vi "LakeShore218_01_Main.vi"() -> ()   [LabVIEW 2019]
uses:
  LakeShore218_Global.vi
panel:
  in  "onoff_ch8":enum16{"Off", "On"}(ring)
  in  "onoff_ch7":enum16{"Off", "On"}(ring)
  in  "onoff_ch6":enum16{"Off", "On"}(ring)
  in  "onoff_ch5":enum16{"Off", "On"}(ring)
  in  "onoff_ch4":enum16{"Off", "On"}(ring)
  in  "onoff_ch3":enum16{"Off", "On"}(ring)
  in  "onoff_ch2":enum16{"Off", "On"}(ring)
  in  "onoff_ch1":enum16{"Off", "On"}(ring)
  out "status_rec":bool=TRUE caption="Logging Status"
  out "Last Measured":timestamp format="%<%Y-%m-%d %H:%M:%S>T"
  out "Chart":waveform(dbl)[](graph)=[{"t0"=timestamp(3753816869.0379753 s since 1904-01-01), "dt"=1.0, "Y"=[1006.8], "attributes"=variant("NI_ChannelName"=variant(string "Buffle Top"))}, {"t0"=timestamp(3753816869.0379753 s since 1904-01-01), "dt"=1.0, "Y"=[1008.0], "attributes"=variant("NI_ChannelName"=variant(string "Buffle Bottom"))}, {"t0"=timestamp(3753816869.0379753 s since 1904-01-01), "dt"=1.0, "Y"=[1008.9], "attributes"=variant("NI_ChannelName"=variant(string "Seperator Top"))}, {"t0"=timestamp(3753816869.0379753 s since 1904-01-01), "dt"=1.0, "Y"=[84.7], "attributes"=variant("NI_ChannelName"=variant(string "Seperator Bottom"))}, {"t0"=timestamp(3753816869.0379753 s since 1904-01-01), "dt"=1.0, "Y"=[1009.7], "attributes"=variant("NI_ChannelName"=variant(string "Heat-Ex Top"))}, {"t0"=timestamp(3753816869.0379753 s since 1904-01-01), "dt"=1.0, "Y"=[1017.1], "attributes"=variant("NI_ChannelName"=variant(string "Heat-Ex Bottom"))}, {"t0"=timestamp(3753816869.0379753 s since 1904-01-01), "dt"=1.0, "Y"=[1020.8], "attributes"=variant("NI_ChannelName"=variant(string "Ann-Plate Bar"))}, {"t0"=timestamp(3753816869.0379753 s since 1904-01-01), "dt"=1.0, "Y"=[1015.3], "attributes"=variant("NI_ChannelName"=variant(string "Ann-Plate Top"))}]
  in  "Interval":u32=1000
  out "status":bool=TRUE
  out "value_array":dbl[](array[numeric]) caption="Last Readings" format="%.1f"
  in  "stop":bool
  in  "VISA":refnum<visa-resource-name>="GPIB0::2::INSTR"
  # "LakeShore218 #01: Fridge Temperature"
  # "ms"
  # "W"
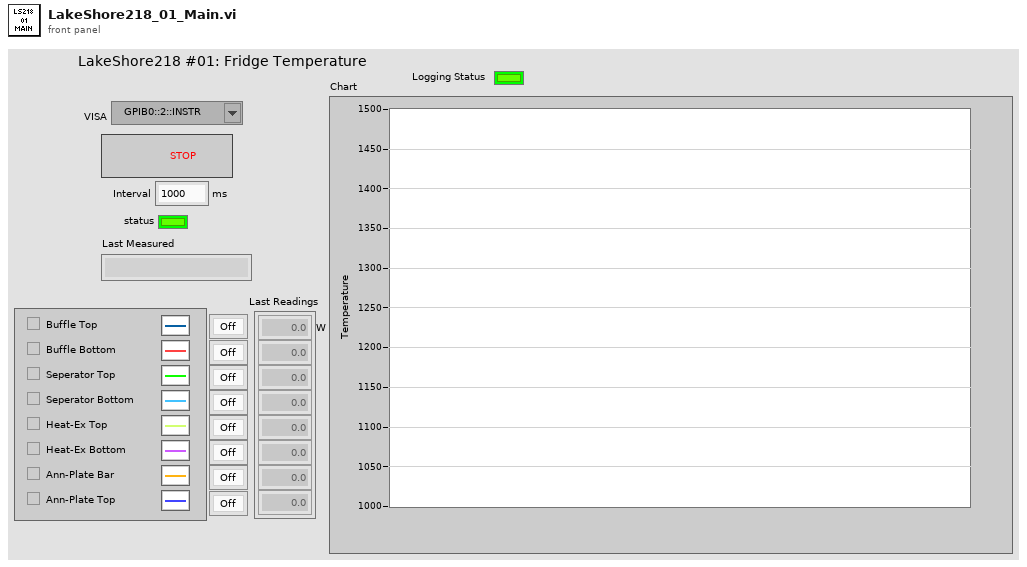
[diagram p1: front panel]
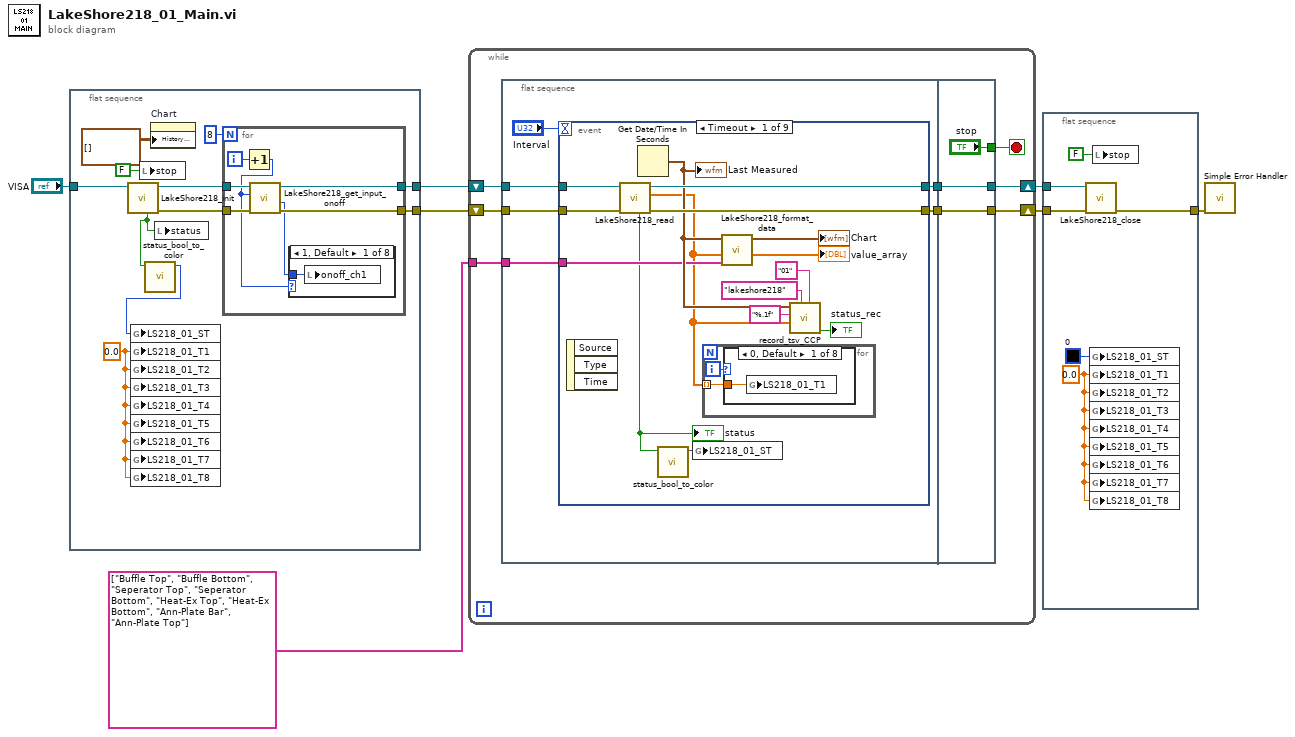
[diagram p0: block diagram]
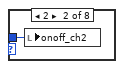
[diagram p2: hidden frame]
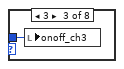
[diagram p3: hidden frame]
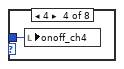
[diagram p4: hidden frame]
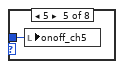
[diagram p5: hidden frame]
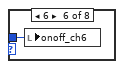
[diagram p6: hidden frame]
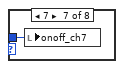
[diagram p7: hidden frame]
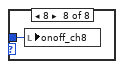
[diagram p8: hidden frame]
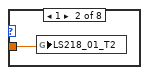
[diagram p9: hidden frame]
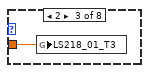
[diagram p10: hidden frame]
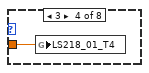
[diagram p11: hidden frame]
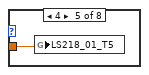
[diagram p12: hidden frame]
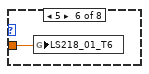
[diagram p13: hidden frame]
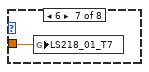
[diagram p14: hidden frame]
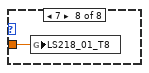
[diagram p15: hidden frame]
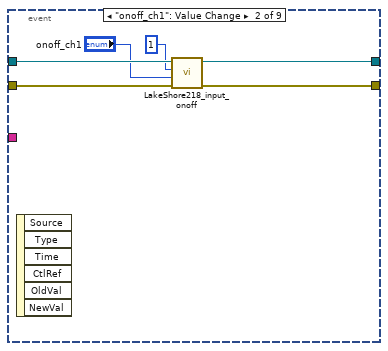
[diagram p16: hidden frame]
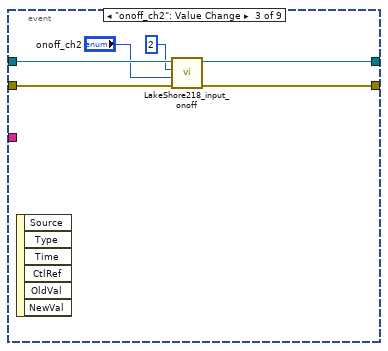
[diagram p17: hidden frame]
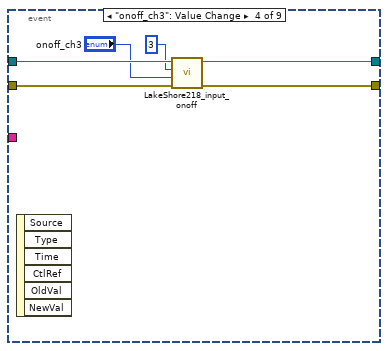
[diagram p18: hidden frame]
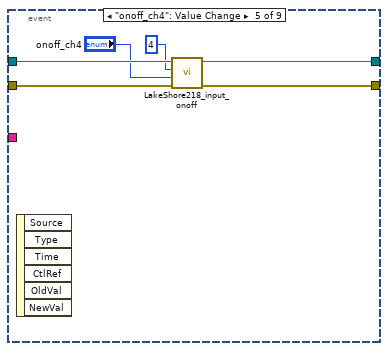
[diagram p19: hidden frame]
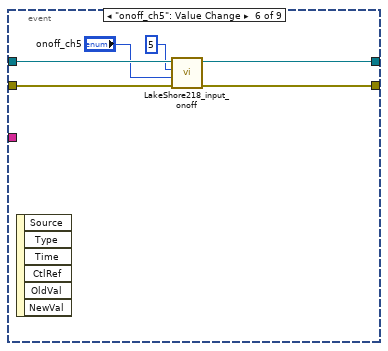
[diagram p20: hidden frame]
diagram:
  n1 = flat-sequence {
    tunnel: [w9] -> w7
    tunnel: [w10] -> w6
    tunnel: "VISA" -> [w18]
    frame #0 {
      w13 = 0.0 ("LS218_01_T1")
      n2 = call "LakeShore218_init.vi"("VISA in"=w18) -> ("error out"=w11:errorcluster, "VISA out"=w12:refnum<visa-resource-name>, "status"=w15:bool)  [unwired: 8 in]
      n3 = global write "LakeShore218_Global.vi" "LS218_01_T1"(w13) -> ()
      n4 = global write "LakeShore218_Global.vi" "LS218_01_T2"(w13) -> ()
      n5 = global write "LakeShore218_Global.vi" "LS218_01_T3"(w13) -> ()
      n6 = global write "LakeShore218_Global.vi" "LS218_01_T4"(w13) -> ()
      n7 = global write "LakeShore218_Global.vi" "LS218_01_T5"(w13) -> ()
      n8 = global write "LakeShore218_Global.vi" "LS218_01_T6"(w13) -> ()
      n9 = global write "LakeShore218_Global.vi" "LS218_01_T7"(w13) -> ()
      n10 = global write "LakeShore218_Global.vi" "LS218_01_T8"(w13) -> ()
      n11 = local write "stop"(FALSE ("stop")) -> ()
      n12 = call "status_bool_to_color.vi"("status_bool_1"=w15) -> ("status_color"=w14:u32)  [unwired: 10 in]
      n13 = global write "LakeShore218_Global.vi" "LS218_01_ST"(w14) -> ()
      n14 = property on="Chart" class="WFChart (strict)"("History Data"=waveform(dbl)[][] []) -> ()  [unwired: 2 in, 2 out]
      n15 = local write "status"(w15) -> ()
      n16 = for {
        N: 8 -> [_]
        tunnel: w12 -> [w25]
        tunnel: w11 -> [w24]
        tunnel: [w23] -> w10
        tunnel: [w22] -> w9
        i -> [w21]
        n17 = Increment(x=w21) -> (x+1=w20:i32)
        n18 = call "LakeShore218_get_input_onoff.vi"("error in"=w24, "channel"=w20, "VISA in"=w25) -> ("error out"=w22:errorcluster, "onoff"=w19:enum16{"Off", "On"}, "VISA out"=w23:refnum<visa-resource-name>)  [unwired: 5 in, 1 out]
        n19 = case shown="1, Default" w20 {
          tunnel: w19 -> [w26 w27 w28 w29 w30 w31 w32 w33]
          frame 1, Default {
            n20 = local write "onoff_ch1"(w26) -> ()
          }
          frame 2 {
            n21 = local write "onoff_ch2"(w27) -> ()
          }
          frame 3 {
            n22 = local write "onoff_ch3"(w28) -> ()
          }
          frame 4 {
            n23 = local write "onoff_ch4"(w29) -> ()
          }
          frame 5 {
            n24 = local write "onoff_ch5"(w30) -> ()
          }
          frame 6 {
            n25 = local write "onoff_ch6"(w31) -> ()
          }
          frame 7 {
            n26 = local write "onoff_ch7"(w32) -> ()
          }
          frame 8 {
            n27 = local write "onoff_ch8"(w33) -> ()
          }
        }
      }
    }
  }
  n28 = while {
    shift-right: [w39] -> w4
    shift-left: w6 -> [w40]
    shift-right: [w38] -> w3
    shift-left: w7 -> [w41]
    tunnel: string[] ["Buffle Top", "Buffle Bottom", "Seperator Top", "Seperator Bottom", "Heat-Ex Top", "Heat-Ex Bottom", "Ann-Plate Bar", "Ann-Plate Top"] ("format_array") -> [w35]
    stop <- w34 stop-if-true
    n29 = flat-sequence {
      tunnel: w41 -> [w47]
      tunnel: w40 -> [w46]
      tunnel: [w45] -> w37
      tunnel: [w44] -> w36
      tunnel: w35 -> [w43]
      tunnel: [w122] -> w38
      tunnel: [w123] -> w39
      tunnel: w37 -> [w123]
      tunnel: w36 -> [w122]
      tunnel: ["stop"] -> w34
      frame #0 {
        n30 = event shown="[0] Timeout" {
          selector: _ -> [_ _ _ _ _ _ _ _ _]
          dyn-events: _ -> [_ _ _ _ _ _ _ _ _]
          timeout: "Interval" -> [_ _ _ _ _ _ _ _ _]
          tunnel: w47 -> [w62 w76 w82 w88 w94 w100 w106 w112 w118]
          tunnel: w46 -> [w61 w78 w84 w90 w96 w102 w108 w114 w120]
          tunnel: [w60 w77 w83 w89 w95 w101 w107 w113 w119] -> w45
          tunnel: [w59 w75 w81 w87 w93 w99 w105 w111 w117] -> w44
          tunnel: w43 -> [w52 _ _ _ _ _ _ _ _]
          event Timeout {
            n31 = event-data() -> ()  [unwired: 1 in, 3 out]
            n32 = call "LakeShore218_read.vi"("error in"=w62, "VISA in"=w61) -> ("error out"=w59:errorcluster, "value_array"=w48:dbl[], "VISA out"=w60:refnum<visa-resource-name>, "status"=w50:bool)  [unwired: 6 in]
            "status" <- w50
            n33 = Get Date/Time In Seconds() -> (seconds since 1Jan1904=w56:timestamp)
            "Last Measured" <- w56
            n34 = call "status_bool_to_color.vi"("status_bool_1"=w50) -> ("status_color"=w49:u32)  [unwired: 10 in]
            n35 = global write "LakeShore218_Global.vi" "LS218_01_ST"(w49) -> ()
            n36 = for {
              tunnel: w48 -> [w63] mode=indexing
              i -> [w64]
              n37 = case shown="0, Default" w64 {
                tunnel: w63 -> [w65 w66 w67 w68 w69 w70 w71 w72]
                frame 0, Default {
                  n38 = global write "LakeShore218_Global.vi" "LS218_01_T1"(w65) -> ()
                }
                frame 1 {
                  n39 = global write "LakeShore218_Global.vi" "LS218_01_T2"(w66) -> ()
                }
                frame 2 {
                  n40 = global write "LakeShore218_Global.vi" "LS218_01_T3"(w67) -> ()
                }
                frame 3 {
                  n41 = global write "LakeShore218_Global.vi" "LS218_01_T4"(w68) -> ()
                }
                frame 4 {
                  n42 = global write "LakeShore218_Global.vi" "LS218_01_T5"(w69) -> ()
                }
                frame 5 {
                  n43 = global write "LakeShore218_Global.vi" "LS218_01_T6"(w70) -> ()
                }
                frame 6 {
                  n44 = global write "LakeShore218_Global.vi" "LS218_01_T7"(w71) -> ()
                }
                frame 7 {
                  n45 = global write "LakeShore218_Global.vi" "LS218_01_T8"(w72) -> ()
                }
              }
            }
            n46 = call "LakeShore218_format_data.vi"("name_array"=w52, "value_array"=w48, "time"=w56) -> ("value_array_out"=→"value_array":dbl[], "waveform_array"=→"Chart":waveform(dbl)[])  [unwired: 7 in]
            n47 = call "record_tsv_CCP.vi"("file_name"="01", "folder_name"="lakeshore218", "value_array"=w48, "format"="%.1f", "time"=w56) -> ("status"=→"status_rec":bool)  [unwired: 5 in, 1 out]
          }
          event "onoff_ch1": Value Change {
            n48 = event-data() -> ()  [unwired: 1 in, 6 out]
            n49 = call "LakeShore218_input_onoff.vi"("error in"=w76, "onoff"="onoff_ch1", "channel"=i8 1, "VISA in"=w78) -> ("error out"=w75:errorcluster, "VISA out"=w77:refnum<visa-resource-name>)  [unwired: 5 in, 1 out]
          }
          event "onoff_ch2": Value Change {
            n50 = event-data() -> ()  [unwired: 1 in, 6 out]
            n51 = call "LakeShore218_input_onoff.vi"("error in"=w82, "onoff"="onoff_ch2", "channel"=i8 2, "VISA in"=w84) -> ("error out"=w81:errorcluster, "VISA out"=w83:refnum<visa-resource-name>)  [unwired: 5 in, 1 out]
          }
          event "onoff_ch3": Value Change {
            n52 = event-data() -> ()  [unwired: 1 in, 6 out]
            n53 = call "LakeShore218_input_onoff.vi"("error in"=w88, "onoff"="onoff_ch3", "channel"=i8 3, "VISA in"=w90) -> ("error out"=w87:errorcluster, "VISA out"=w89:refnum<visa-resource-name>)  [unwired: 5 in, 1 out]
          }
          event "onoff_ch4": Value Change {
            n54 = event-data() -> ()  [unwired: 1 in, 6 out]
            n55 = call "LakeShore218_input_onoff.vi"("error in"=w94, "onoff"="onoff_ch4", "channel"=i8 4, "VISA in"=w96) -> ("error out"=w93:errorcluster, "VISA out"=w95:refnum<visa-resource-name>)  [unwired: 5 in, 1 out]
          }
          event "onoff_ch5": Value Change {
            n56 = event-data() -> ()  [unwired: 1 in, 6 out]
            n57 = call "LakeShore218_input_onoff.vi"("error in"=w100, "onoff"="onoff_ch5", "channel"=i8 5, "VISA in"=w102) -> ("error out"=w99:errorcluster, "VISA out"=w101:refnum<visa-resource-name>)  [unwired: 5 in, 1 out]
          }
          event "onoff_ch6": Value Change {
            n58 = event-data() -> ()  [unwired: 1 in, 6 out]
            n59 = call "LakeShore218_input_onoff.vi"("error in"=w106, "onoff"="onoff_ch6", "channel"=i8 6, "VISA in"=w108) -> ("error out"=w105:errorcluster, "VISA out"=w107:refnum<visa-resource-name>)  [unwired: 5 in, 1 out]
          }
          event "onoff_ch7": Value Change {
            n60 = event-data() -> ()  [unwired: 1 in, 6 out]
            n61 = call "LakeShore218_input_onoff.vi"("error in"=w112, "onoff"="onoff_ch7", "channel"=i8 7, "VISA in"=w114) -> ("error out"=w111:errorcluster, "VISA out"=w113:refnum<visa-resource-name>)  [unwired: 5 in, 1 out]
          }
          event "onoff_ch8": Value Change {
            n62 = event-data() -> ()  [unwired: 1 in, 6 out]
            n63 = call "LakeShore218_input_onoff.vi"("error in"=w118, "onoff"="onoff_ch8", "channel"=i8 8, "VISA in"=w120) -> ("error out"=w117:errorcluster, "VISA out"=w119:refnum<visa-resource-name>)  [unwired: 5 in, 1 out]
          }
        }
      }
      frame #1 {
      }
    }
  }
  n64 = flat-sequence {
    tunnel: w4 -> [w129]
    tunnel: w3 -> [w128]
    tunnel: [w127] -> w2
    frame #0 {
      w125 = 0.0 ("LS218_01_T1")
      n65 = call "LakeShore218_close.vi"("error in"=w128, "VISA in"=w129) -> ("error out"=w127:errorcluster)  [unwired: 9 in]
      n66 = global write "LakeShore218_Global.vi" "LS218_01_ST"(u32 0 ("LS218_01_ST")) -> ()
      n67 = global write "LakeShore218_Global.vi" "LS218_01_T1"(w125) -> ()
      n68 = global write "LakeShore218_Global.vi" "LS218_01_T2"(w125) -> ()
      n69 = global write "LakeShore218_Global.vi" "LS218_01_T3"(w125) -> ()
      n70 = global write "LakeShore218_Global.vi" "LS218_01_T4"(w125) -> ()
      n71 = global write "LakeShore218_Global.vi" "LS218_01_T5"(w125) -> ()
      n72 = global write "LakeShore218_Global.vi" "LS218_01_T6"(w125) -> ()
      n73 = global write "LakeShore218_Global.vi" "LS218_01_T7"(w125) -> ()
      n74 = global write "LakeShore218_Global.vi" "LS218_01_T8"(w125) -> ()
      n75 = local write "stop"(FALSE ("stop")) -> ()
    }
  }
  n76 = call <vilib>:"Simple Error Handler.vi"("error in (no error)"=w2) -> ()  [unwired: 4 in, 5 out]
